vi "Get FPGA Paths.vi"(6 "Filter Customized (T)":bool=TRUE, 8 "error in (no error)":errorcluster) -> (0 "error out":errorcluster, 3 "FPGA Personality File Paths":path[](array[path]))   [LabVIEW 2021, in "Personality.lvlib"]
doc: "Gets all the FPGA personality file paths. You could filter the customized FPGA personality file with the Customized tag as true."
uses:
  <vilib>/myRIO/Common/FPGA Personality Framework/Personality.lvlib
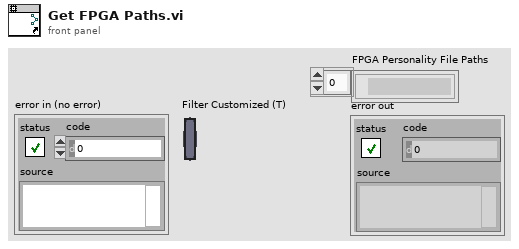
[diagram p1: front panel]
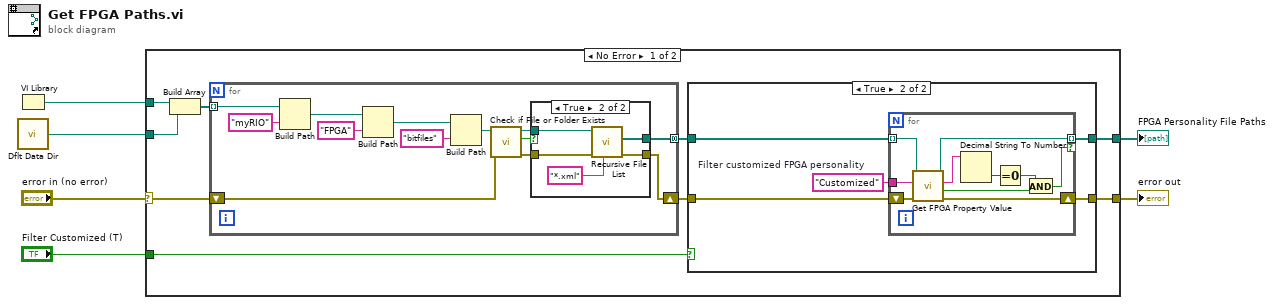
[diagram p0: block diagram]
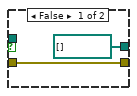
[diagram p3: hidden frame]
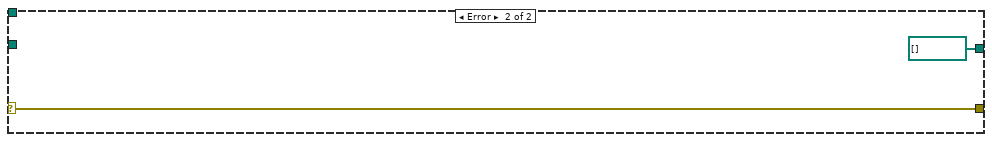
[diagram p4: hidden frame]
diagram:
  n1 = VI Library() -> (path=w6:path)
  n2 = call <vilib>:"Dflt Data Dir.vi"() -> ("App:Default Data Directory"=w4:path)
  n3 = case shown="No Error" "error in (no error)" {
    selector: "error in (no error)" -> [w14 w54]
    tunnel: w6 -> [w15 _]
    tunnel: w4 -> [w13 _]
    tunnel: "Filter Customized (T)" -> [w12 _]
    tunnel: [w11 path[] [] ("All Files in Dir")] -> w2
    tunnel: [w10 w54] -> w1
    frame No Error {
      n4 = Build Array(w15, w13) -> (w9:path[])
      n5 = for {
        tunnel: [w40] -> w8 mode=concatenating
        shift-right: [w33] -> w7
        shift-left: w14 -> [w34]
        tunnel: w9 -> [w39] mode=indexing
        n6 = Build Path(base path=w39, name or relative path="myRIO") -> (appended path=w45:path)
        n7 = Build Path(base path=w45, name or relative path="FPGA") -> (appended path=w44:path)
        n8 = Build Path(base path=w44, name or relative path="bitfiles") -> (appended path=w38:path)
        n9 = call <vilib>:"Check if File or Folder Exists.vi"("error in (no error)"=w34, "path"=w38) -> ("error out"=w35:errorcluster, "file or folder exists?"=w36:bool, "dup path"=w37:path)  [unwired: 7 in]
        n10 = case shown="True" w36 {
          tunnel: [path[] [] ("All Files in Dir") w51] -> w40
          tunnel: w37 -> [_ w50]
          tunnel: w35 -> [w46 w49]
          tunnel: [w46 w48] -> w33
          frame False {
          }
          frame True {
            n11 = call <vilib>:"Recursive File List.vi"("pattern"="*.xml", "error in (no error)"=w49, "Folder Path"=w50) -> ("error out"=w48:errorcluster, "All Files in Dir"=w51:path[])  [unwired: 4 in, 3 out]
          }
        }
      }
      n12 = case shown="True" w12 {
        tunnel: w8 -> [w17 w20]
        tunnel: [w17 w21] -> w11
        tunnel: w7 -> [w16 w19]
        tunnel: [w16 w18] -> w10
        frame False {
        }
        frame True {
          w22 = "Customized"  # Filter customized FPGA personality
          n13 = for {
            shift-right: [w31] -> w18
            shift-left: w19 -> [w32]
            tunnel: w22 -> [w28]
            tunnel: [w30] -> w21 mode=indexing if=w25
            tunnel: w20 -> [w29] mode=indexing
            n14 = call <vilib>:"Get FPGA Property Value.vi"("error in (no error)"=w32, "Property Name"=w28, "FPGA Personality File Path"=w29) -> ("error out"=w31:errorcluster, "Found?"=w24:bool, "Property Value"=w27:string, "Duplicated FPGA Personality File Path"=w30:path)  [unwired: 5 in]
            n15 = Decimal String To Number(string=w27) -> (number=w26:i32)  [unwired: 2 in, 1 out]
            n16 = Equal To 0?(x=w26) -> (x = 0?=w23:bool)
            n17 = And(x=w23, y=w24) -> (x .and. y?=w25:bool)
          }
        }
      }
    }
    frame Error {
    }
  }
  "error out" <- w1
  "FPGA Personality File Paths" <- w2
